vi "Write Current Cell.vi"(8 "error in":errorcluster, 10 "Current Cell":i32, 11 "PAS Data in":refnum<class "PAS Data.lvclass">) -> (0 "error out":errorcluster, 3 "PAS Data out":refnum<class "PAS Data.lvclass">)   [LabVIEW 2017, in "PAS Library.lvlib" / "PAS Data.lvclass"]
uses:
  PAS Data.lvclass
  PAS Data.lvclass/PAS Data.ctl
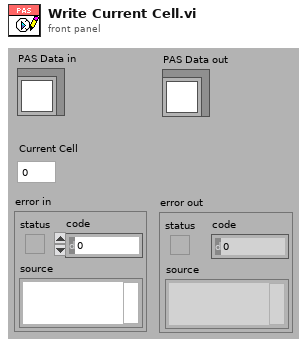
[diagram p1: front panel]
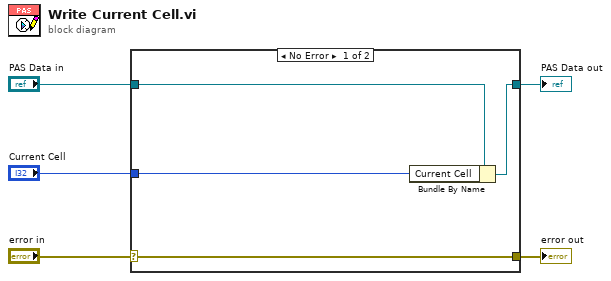
[diagram p0: block diagram]
diagram:
  n1 = case shown="No Error" "error in" {
    selector: "error in" -> [w9 w10]
    tunnel: [w9 w10] -> w4
    tunnel: [w7 w11] -> w2
    tunnel: "PAS Data in" -> [w8 w11]
    tunnel: "Current Cell" -> [w6 _]
    frame No Error {
      n2 = Bundle By Name(cluster=w8, "Current Cell"=w6) -> (w7:refnum<class "PAS Data.lvclass">)
    }
    frame Error {
    }
  }
  "error out" <- w4
  "PAS Data out" <- w2
